vi "Copy .LLB to NI VeriStand dir.vi"(5 "Files Generated by Build":path[](array[path]), 6 "Top Level/Always Included VIs":path[](array[path]), 7 "Destination Path":path, 8 "error in (no error)":errorcluster, 9 "Target Name":string, 10 "Build Specification Name":string, 11 "Project Path":path) -> (0 "error out":errorcluster)   [LabVIEW 2024]
doc: "This VI is called after each run of a build specification. The VI will copy the generated LLB (Engine or System Explorer) into the VeriStand Custom Device folder (...\\Documents\\National Instruments\\NI VeriStand 2013...)."
uses:
  NationalInstruments.VeriStand
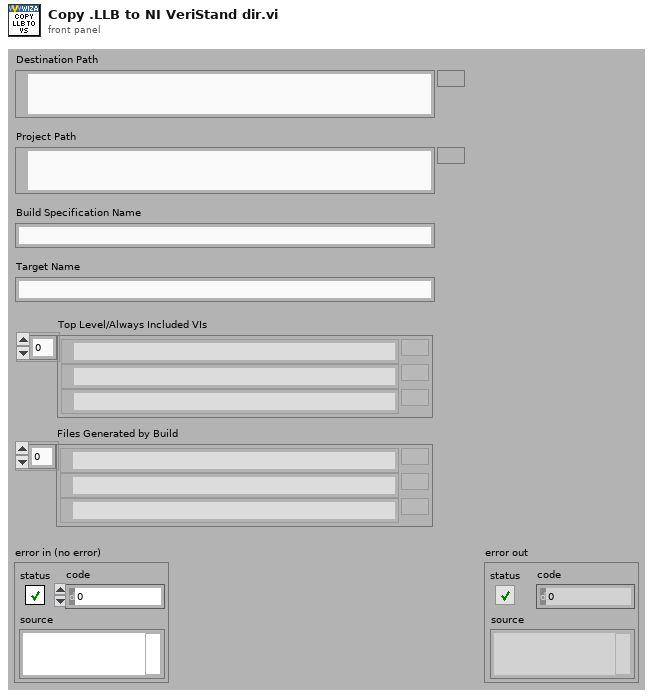
[diagram p1: front panel]
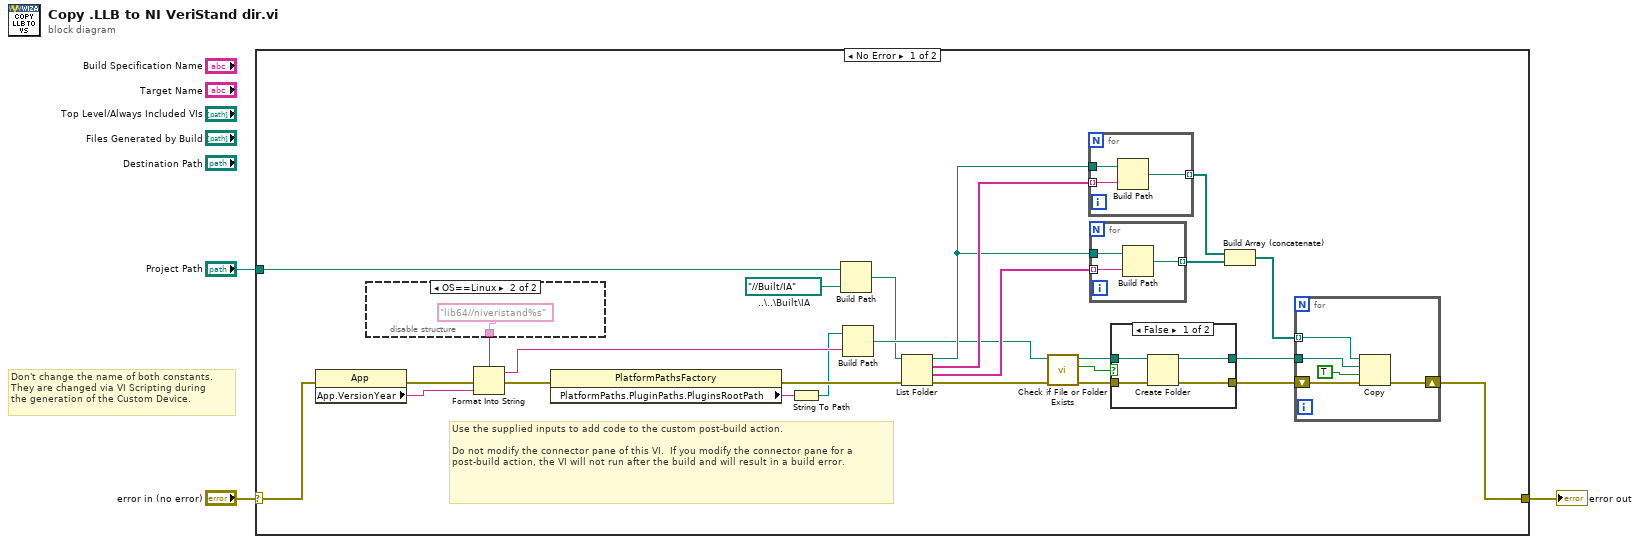
[diagram p0: block diagram]
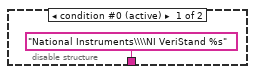
[diagram p2: hidden frame]
diagram:
  # "Don't change the name of both constants.\nThey are changed via VI Scripting during\nthe generation of the Custom Device."
  n1 = case shown="No Error" "error in (no error)" {
    selector: "error in (no error)" -> [w13 w49]
    tunnel: [w15 w49] -> w1
    tunnel: "Project Path" -> [w12 _]
    frame No Error {
      w8 = path "../../Built/IA"  # ..\..\Built\IA
      # "Use the supplied inputs to add code to the custom post-build action.\n\nDo not modify the connector pane of this VI.  If you modify the connector pane for a post-build action, the VI will not run after the build and will result in a build error."
      n2 = property class="App"(error in=w13) -> (error out=w18:errorcluster, "App.VersionYear"=w17:string)  [unwired: 1 in, 1 out]
      n3 = disable-structure shown="OS==Linux" {
        disable-tunnel: ["National Instruments\\\\NI VeriStand %s" ("name or relative path") "lib64//niveristand%s" ("name or relative path")] -> w16
        frame condition #0 (active) {
        }
        frame condition #1 {
        }
      }
      n4 = Format Into String(format string=w16, error in=w18, w17) -> (resulting string=w19:string, error out=w7:errorcluster)  [unwired: 1 in]
      n5 = property class="PlatformPathsFactory"(error in=w7) -> (error out=w6:errorcluster, "PlatformPaths.PluginPaths.PluginsRootPath"=w5:string)  [unwired: 1 in, 1 out]
      n6 = String To Path(string=w5) -> (path=w4:path)
      n7 = Build Path(base path=w12, name or relative path=w8) -> (appended path=w9:path)
      n8 = Build Path(base path=w4, name or relative path=w19) -> (appended path=w14:path)
      n9 = List Folder(path=w9, error in=w6) -> (path out=w22:path, filenames=w29:string[], folder names=w23:string[], error out=w20:errorcluster)  [unwired: 2 in]
      n10 = call <vilib>:"Check if File or Folder Exists.vi"("error in (no error)"=w20, "path"=w14) -> ("error out"=w24:errorcluster, "file or folder exists?"=w26:bool, "dup path"=w25:path)  [unwired: 7 in]
      n11 = for {
        tunnel: w29 -> [w47] mode=indexing
        tunnel: w22 -> [w48]
        tunnel: [w46] -> w28 mode=indexing
        n12 = Build Path(base path=w48, name or relative path=w47) -> (appended path=w46:path)
      }
      n13 = for {
        tunnel: w23 -> [w44] mode=indexing
        tunnel: w22 -> [w45]
        tunnel: [w43] -> w21 mode=indexing
        n14 = Build Path(base path=w45, name or relative path=w44) -> (appended path=w43:path)
      }
      n15 = case shown="False" w26 {
        tunnel: w25 -> [w35 w37]
        tunnel: w24 -> [w34 w36]
        tunnel: [w33 w37] -> w11
        tunnel: [w32 w36] -> w10
        frame False {
          n16 = Create Folder(path (use dialog)=w35, error in=w34) -> (created path=w33:path, error out=w32:errorcluster)  [unwired: 1 in, 1 out]
        }
        frame True {
        }
      }
      n17 = Build Array (concatenate)(w28, w21) -> (w27:path[])
      n18 = for {
        tunnel: w27 -> [w39] mode=indexing
        shift-right: [w40] -> w15
        shift-left: w10 -> [w41]
        tunnel: w11 -> [w38]
        n19 = Copy(8:w41, 9:TRUE ("overwrite (F)"), 10:w38, 11:w39) -> (0:w40:errorcluster)  [unwired: 1 in, 2 out]
      }
    }
    frame Error {
    }
  }
  "error out" <- w1
